vi "Give log reference if debugging.vi"(7 "application ref":refnum<vi>, 8 "error in (no error)":errorcluster, 11 "log reference in":refnum<vi>) -> (0 "error out":errorcluster, 3 "log reference out":refnum<vi>, 4 "is executable?":bool)   [LabVIEW 2012]
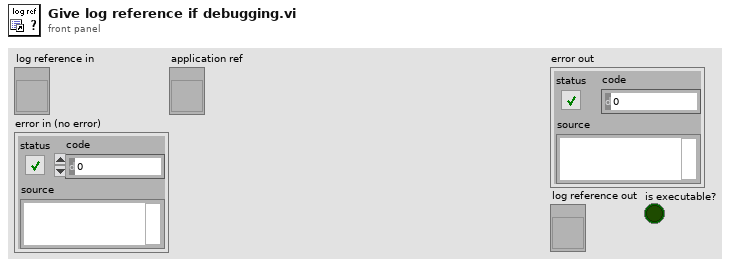
[diagram p1: front panel]
types:
  T1 = enum32{"invalid app kind", "Development System", "Run Time System", "Student Edition", "Embedded LabVIEW", "Evaluation", "Custom"}
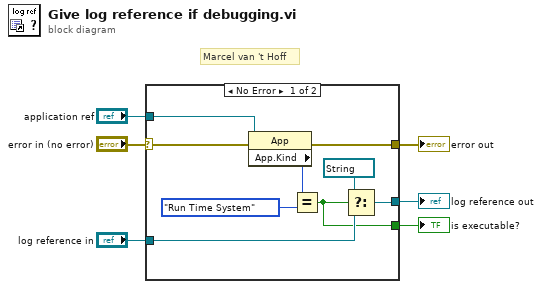
[diagram p0: block diagram]
diagram:
  # "Marcel van 't Hoff"
  n1 = case shown="No Error" "error in (no error)" {
    selector: "error in (no error)" -> [w8 w17]
    tunnel: "log reference in" -> [w12 w16]
    tunnel: [w11 w17] -> w5
    tunnel: [w10 w16] -> w4
    tunnel: [w9 _] -> w3
    tunnel: "application ref" -> [w7 _]
    frame No Error {
      n2 = property class="App"(reference=w7, error in=w8) -> (error out=w11:errorcluster, "App.Kind"=w13:T1)  [unwired: 1 out]
      n3 = Equal?(x=w13, y=T1."Run Time System" ("Application:Kind")) -> (x = y?=w9:bool)
      n4 = Select(t=refnum<vi> refnum, s=w9, f=w12) -> (s? t:f=w10:refnum<vi>)
    }
    frame Error {
    }
  }
  "error out" <- w5
  "log reference out" <- w4
  "is executable?" <- w3
